vi "CreateFile.vi"() -> (0 "error out":errorcluster, 2 "Date/Time":string, 3 "Byte Stream File out":refnum<file>)   [LabVIEW 2017]
uses:
  <vilib>/Rock Robotics/Network Tables/NT Read String.vi
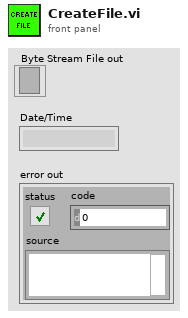
[diagram p1: front panel]
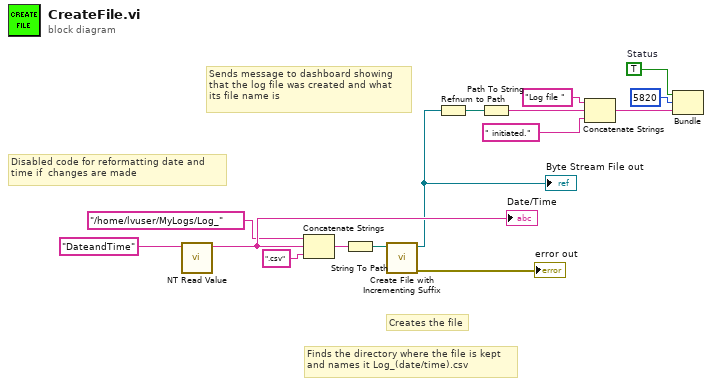
[diagram p0: block diagram]
diagram:
  w10 = TRUE  # Status
  # "Finds the directory where the file is kept\nand names it Log_(date/time).csv"
  # "Creates the file"
  # "Sends message to dashboard showing\nthat the log file was created and what \nits file name is"
  # "Disabled code for reformatting date and \ntime if  changes are made"
  n1 = call-poly <vilib>:"NT Read Value.vi"("Name"="DateandTime") -> ("String"=w15:string)  [unwired: 9 in, 1 out]
  "Date/Time" <- w15
  n2 = Concatenate Strings("/home/lvuser/MyLogs/Log_" ("string"), w15, ".csv" ("string")) -> (w7:string)
  n3 = String To Path(string=w7) -> (path=w6:path)
  n4 = call <vilib>:"Create File with Incrementing Suffix.vi"("file path"=w6) -> ("error out"=→"error out":errorcluster, "refnum out"=w13:refnum<file>)  [unwired: 8 in, 1 out]
  "Byte Stream File out" <- w13
  n5 = Refnum to Path(1:w13) -> (0:w4:path)
  n6 = Path To String(path=w4) -> (string=w3:string)
  n7 = Concatenate Strings("Log file " ("Source"), w3, " initiated." ("string")) -> (w12:string)
  n8 = Bundle("Status"=w10, "Code"=u32 5820, w12) -> ()  [unwired: 1 in, 1 out]
